vi "Read AGAINx.vi"(8 "error in (no error)":errorcluster, 11 "AMS TS3472 in":refnum<class "AMS TCS3472.lvclass">) -> (0 "error out":errorcluster, 2 "AGAINx":i32, 3 "AMS TS3472 out":refnum<class "AMS TCS3472.lvclass">)   [LabVIEW 2016, in "AMS TS3472 Light Sensor.lvlib" / "AMS TCS3472.lvclass"]
uses:
  AMS TCS3472.lvclass
  AMS TCS3472.lvclass/AMS TCS3472.ctl
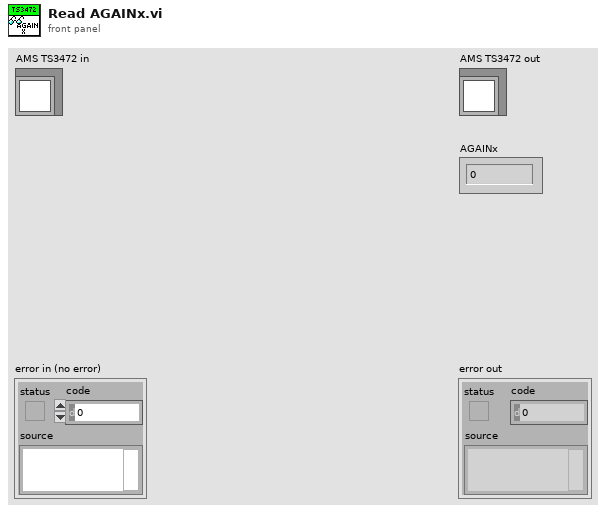
[diagram p1: front panel]
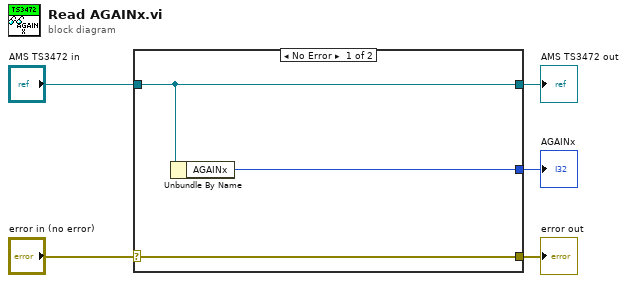
[diagram p0: block diagram]
diagram:
  n1 = case shown="No Error" "error in (no error)" {
    selector: "error in (no error)" -> [w8 w9]
    tunnel: [w8 w9] -> w4
    tunnel: [w7 w10] -> w2
    tunnel: "AMS TS3472 in" -> [w7 w10]
    tunnel: [w6 _] -> w1
    frame No Error {
      n2 = Unbundle By Name(w7) -> ("AGAINx"=w6:i32)
    }
    frame Error {
    }
  }
  "error out" <- w4
  "AMS TS3472 out" <- w2
  "AGAINx" <- w1
